vi "Generate Food Locations.vi"(11 "Num Food":i32=1) -> (3 "Food Array":i32[][](array[numeric]))   [LabVIEW 2014]
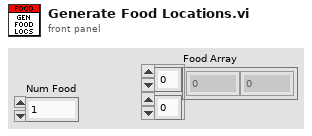
[diagram p1: front panel]
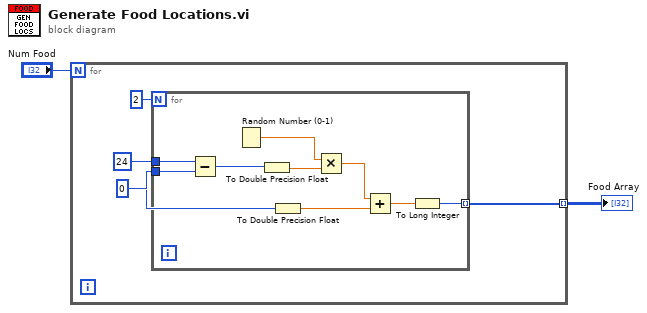
[diagram p0: block diagram]
diagram:
  n1 = for {
    N: "Num Food" -> [_]
    tunnel: [w3] -> w2 mode=indexing
    n2 = for {
      N: 2 -> [_]
      tunnel: 24 ("MAX") -> [w15]
      tunnel: 0 ("MIN") -> [w13]
      tunnel: [w10] -> w3 mode=indexing
      n3 = Subtract(x=w15, y=w13) -> (x-y=w14:i32)
      n4 = Random Number (0-1)() -> (number: 0 to 1=w9:dbl)
      n5 = To Double Precision Float(number=w14) -> (double precision float=w8:dbl)
      n6 = To Double Precision Float(number=w13) -> (double precision float=w12:dbl)
      n7 = Multiply(x=w9, y=w8) -> (x*y=w7:dbl)
      n8 = Add(x=w7, y=w12) -> (x+y=w11:dbl)
      n9 = To Long Integer(number=w11) -> (32bit integer=w10:i32)
    }
  }
  "Food Array" <- w2
